vi "Ctor.vi"(8 "error in (no error)":errorcluster, 11 "InsertionPalettePanel in":refnum<class "InsertionPalettePanel.lvclass">) -> (0 "error out":errorcluster, 3 "InsertionPalettePanel out":refnum<class "InsertionPalettePanel.lvclass">)   [LabVIEW 2020, in "TSnax UI.lvlib" / "InsertionPalettePanel.lvclass"]
uses:
  InsertionPalettePanel.lvclass
  Ref Data.ctl
  StepTypeMenuItem/StepTypeMenuItem.lvclass
  InsertionPalettePanel.lvclass/InsertionPalettePanel.ctl
  <vilib>/IlluminatedG/IG OOPanel/OOPanel/Panel/Panel.lvclass
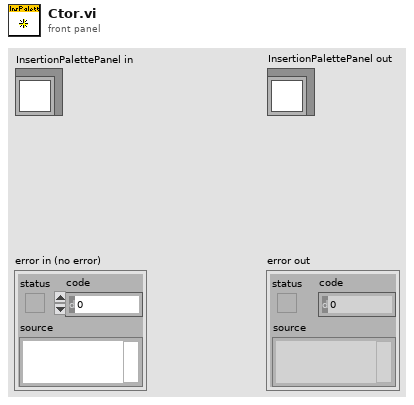
[diagram p1: front panel]
types:
  T1 = typedef "TSnax UI.lvlib/InsertionPalettePanel.lvclass/Ref Data.ctl" = cluster{"Menu Items":map{string, refnum<class "StepTypeMenuItem.lvclass">}}
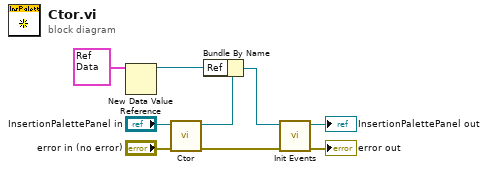
[diagram p0: block diagram]
diagram:
  n1 = New Data Value Reference(data value=T1 {"Menu Items"={}} ("Ref Data")) -> (data value reference=w7:refnum<data-value>)  [unwired: 1 in, 1 out]
  n2 = call-parent "Ctor.vi"("error in (no error)"="error in (no error)", "Panel in"="InsertionPalettePanel in") -> ("error out"=w2:errorcluster, "Panel out"=w6:refnum<class "InsertionPalettePanel.lvclass">)  [unwired: 8 in]
  n3 = Bundle By Name(cluster=w6, "Ref"=w7) -> (w1:refnum<class "InsertionPalettePanel.lvclass">)
  n4 = call "Init Events.vi"("error in (no error)"=w2, "InsertionPalettePanel in"=w1) -> ("error out"=→"error out":errorcluster, "InsertionPalettePanel out"=→"InsertionPalettePanel out":refnum<class "InsertionPalettePanel.lvclass">)  [unwired: 8 in]
